vi "String Test.vi"() -> ()   [LabVIEW 2010]
uses:
  <vilib>/MDSplus/Classes/Data_Class/Scalar_Class/String_Class/String.lvclass
panel:
  out "Equals?":bool
  out "String value out 2":string
  out "String value out":string
  in  "String value in 2":string="String 2"
  in  "String value in":string="String 1"
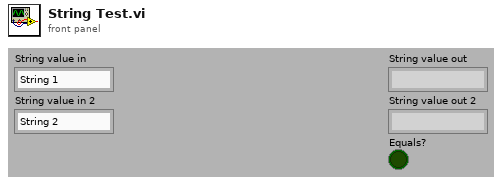
[diagram p1: front panel]
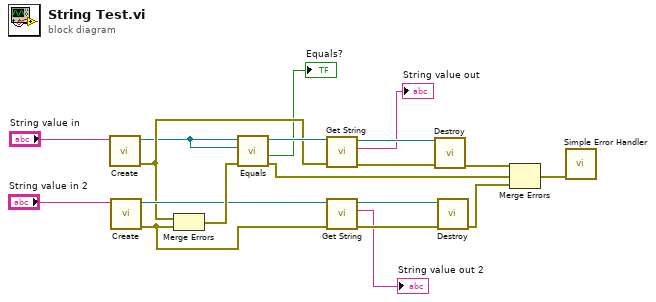
[diagram p0: block diagram]
diagram:
  n1 = call <vilib>:"Create.vi"("String value in"="String value in") -> ("error out"=w14:errorcluster, "String out"=w2:refnum<class "String.lvclass">)  [unwired: 9 in]
  n2 = call <vilib>:"Create.vi"("String value in"="String value in 2") -> ("error out"=w15:errorcluster, "String out"=w16:refnum<class "String.lvclass">)  [unwired: 9 in]
  n3 = Merge Errors(w14, w15) -> (w18:errorcluster)
  n4 = call-dynamic "Equals.vi"("error in (no error)"=w18, "Data in"=w2, "String in"=w2) -> ("error out"=w6:errorcluster, "Equals?"=→"Equals?":bool, "String out"=w17:refnum<class "String.lvclass">)  [unwired: 5 in, 1 out]
  n5 = call-dynamic "Get String.vi"("error in (no error)"=w14, "String in"=w17) -> ("error out"=w13:errorcluster, "String value out"=→"String value out":string, "String out"=w10:refnum<class "String.lvclass">)  [unwired: 7 in]
  n6 = call-dynamic "Get String.vi"("error in (no error)"=w15, "String in"=w16) -> ("error out"=w12:errorcluster, "String value out"=→"String value out 2":string, "String out"=w11:refnum<class "String.lvclass">)  [unwired: 7 in]
  n7 = call-dynamic "Destroy.vi"("error in (no error)"=w13, "String in"=w10) -> ("error out"=w7:errorcluster)  [unwired: 9 in]
  n8 = call-dynamic "Destroy.vi"("error in (no error)"=w12, "String in"=w11) -> ("error out"=w5:errorcluster)  [unwired: 9 in]
  n9 = Merge Errors(w7, w6, w5) -> (w4:errorcluster)
  n10 = call <vilib>:"Simple Error Handler.vi"("error in (no error)"=w4) -> ()  [unwired: 4 in, 5 out]
